vi "testing arm geometry.vi"(11 "arm angle (deg)":dbl(knob) min=-30.0 max=30.0 scale=30.0..-30.0) -> (1 "arm shuttle":cluster{"x":dbl, "y":dbl}={"x"=-9.11895003862225, "y"=13.0}, 3 "stroke max":dbl=17.75)   [LabVIEW 2020]
panel:
  out "angle (PI)":dbl=0.5 format="%.3g"
  out "In Range?":bool
  out "link to arm":cluster{"x":dbl, "y":dbl}={"x"=2.5000000000000004, "y"=16.0}
  out "hook ctr wrt CG":cluster{"x":dbl, "y":dbl}={"x"=4.000000000000003, "y"=46.25}
  in  "robot frame length (in)":dbl=30.0 format="%#_13g"
  in  "testing?":bool
  in  "hook outer diam (in)":dbl=4.0 format="%.3g"
  in  "coords to link (in)":cluster{"x":dbl, "y":dbl}[](array[cluster])=[{"x"=0.0, "y"=9.0}, {"x"=1.5, "y"=0.0}]
  in  "screw link (in)":dbl=12.0 format="%.3g"
  in  "stop":bool
  out "XY Graph":cluster{dbl[], dbl[]}[](graph)=[{[-31.0, -31.0, 31.0, 31.0], [0.0, 66.0, 66.0, 0.0]}, {[-29.0, -29.0, 29.0, 29.0], [0.0, 64.0, 64.0, 0.0]}, {[4.0, 4.000000000000003], [7.0, 46.25]}, {[2.5000000000000004, -9.11895003862225], [16.0, 13.0]}]
  in  "arm coords (in)":cluster{"x":dbl, "y":dbl}[](array[cluster])=[{"x"=0.0, "y"=32.5}, {"x"=0.0, "y"=3.0}, {"x"=0.0, "y"=3.75}]
  in  "screw pin AG (in)":dbl=13.0 format="%.3g"
  in  "shoulder pin back from CG (in)":dbl=4.0 format="%.3g"
  in  "shoulder pin AG (in)":dbl=7.0 format="%.3g"
  in  "Stroke (in)":dbl(slide) scale=0.0..23.0
  in  "height limit HANGAR (in)":dbl=66.0 format="%.3g"
  in  "frame reach limit (in)":dbl=16.0 format="%.3g"
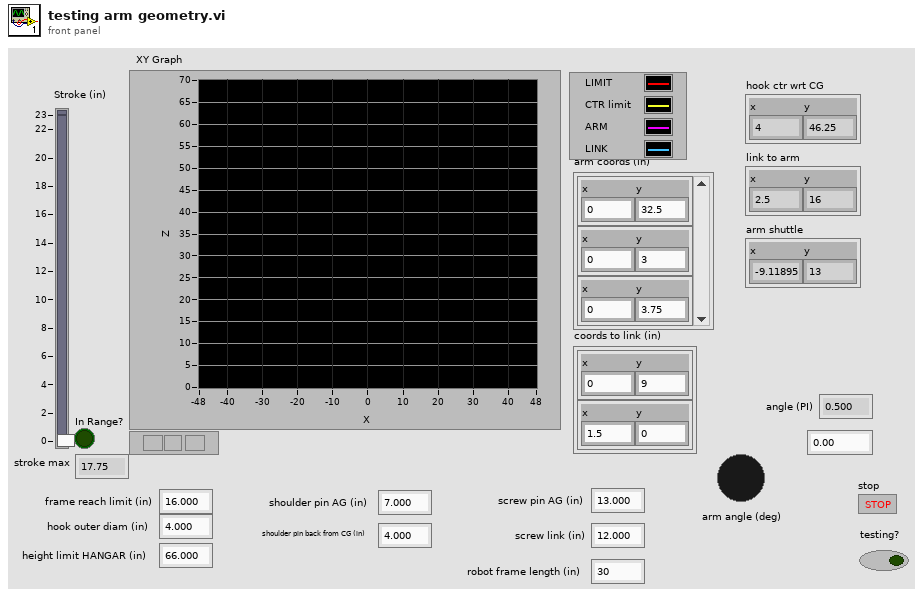
[diagram p1: front panel]
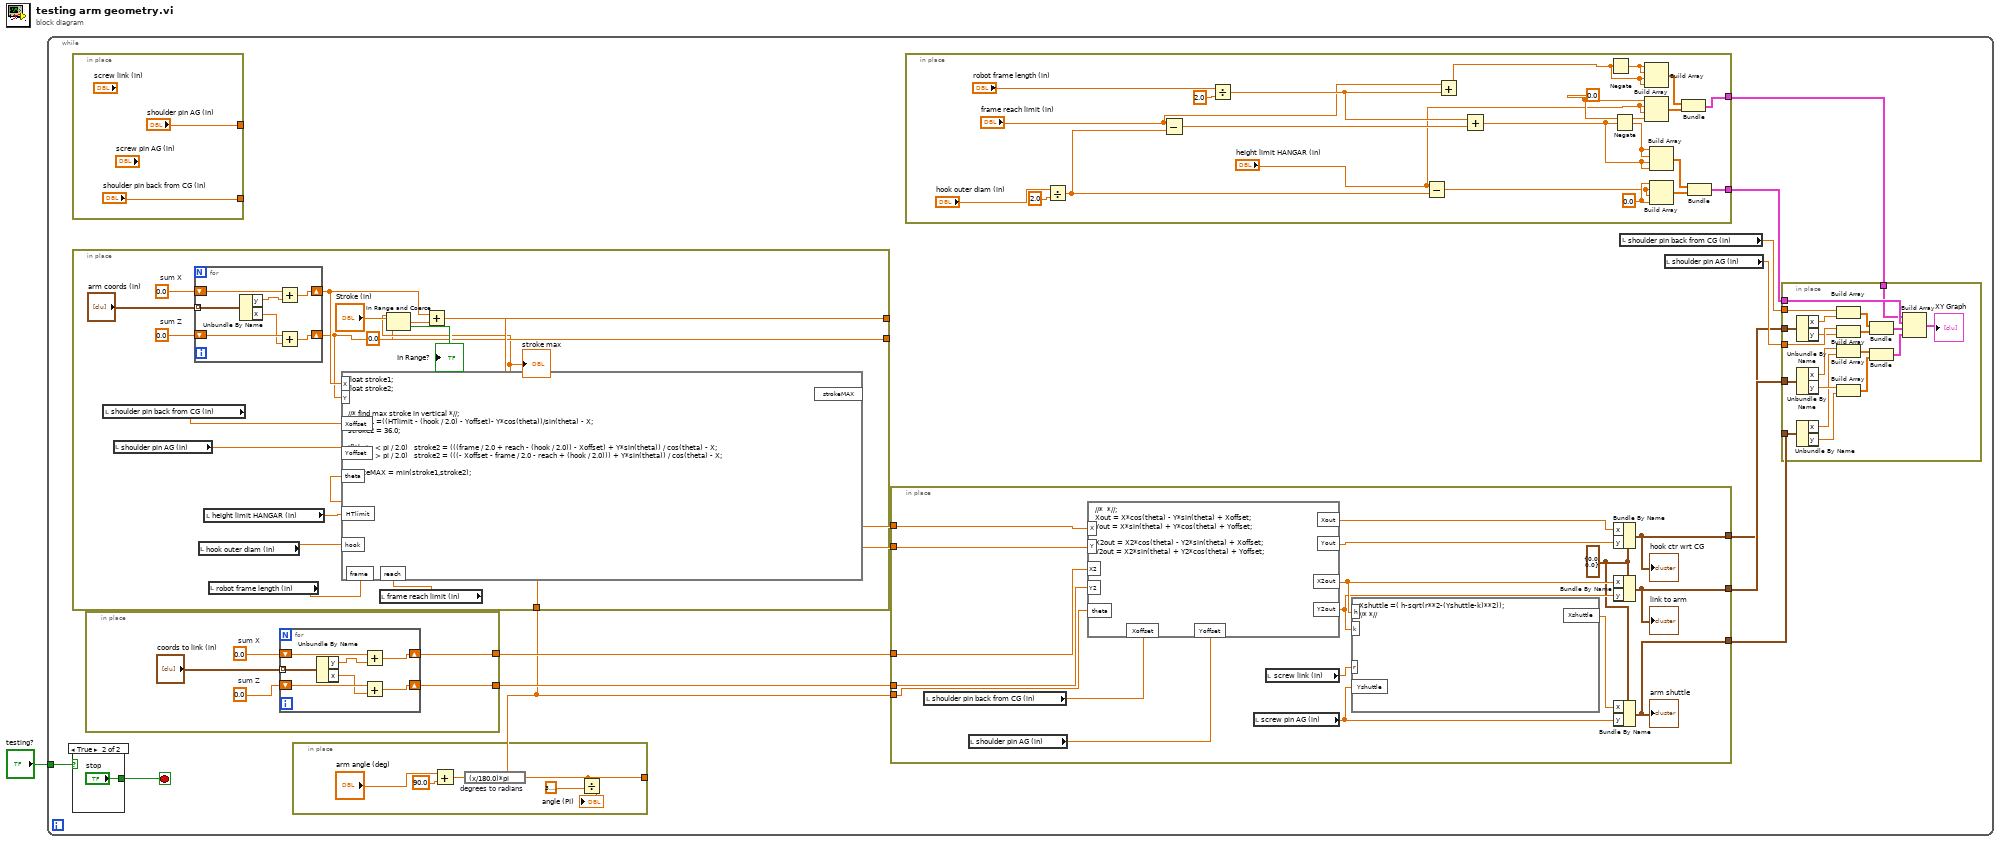
[diagram p0: block diagram]
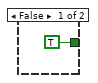
[diagram p2: hidden frame]
diagram:
  n1 = while {
    tunnel: "testing?" -> [w13]
    stop <- w15 stop-if-true
    n2 = in-place {
      in-place-border: ["shoulder pin back from CG (in)"] -> _
      in-place-border: ["shoulder pin AG (in)"] -> _
    }
    n3 = case shown="True" w13 {
      tunnel: [TRUE ("stop") "stop"] -> w15
      frame False {
      }
      frame True {
      }
    }
    n4 = in-place {
      in-place-border: [w64] -> w11
      in-place-border: [w62] -> w12
      w66 = 0.0  # sum X
      w65 = 0.0  # sum Z
      n5 = for {
        tunnel: "coords to link (in)" -> [w73] mode=indexing
        shift-right: [w71] -> w64
        shift-left: w65 -> [w72]
        shift-right: [w70] -> w62
        shift-left: w66 -> [w69]
        n6 = Unbundle By Name(w73) -> ("y"=w68:dbl, "x"=w67:dbl)
        n7 = Add(x=w69, y=w68) -> (x+y=w70:dbl)
        n8 = Add(x=w72, y=w67) -> (x+y=w71:dbl)
      }
    }
    n9 = in-place {
      in-place-border: [w41] -> w2
      n10 = Add(x="arm angle (deg)", y=90.0) -> (x+y=w38:dbl)
      n11 = expression code="(x/180.0)*pi" "degrees to radians"(w38) -> (w41:dbl)
      n12 = Divide(x=w41, y=3.141592653589793) -> (x/y=→"angle (PI)":dbl)
    }
    n13 = in-place {
      in-place-border: [w111] -> w10
      in-place-border: [w105] -> w9
      in-place-border: w2 -> [w103]
      w114 = 0.0  # sum X
      w113 = 0.0  # sum Z
      n14 = local read "shoulder pin back from CG (in)"() -> (w108:dbl)
      n15 = local read "shoulder pin AG (in)"() -> (w107:dbl)
      n16 = for {
        tunnel: "arm coords (in)" -> [w122] mode=indexing
        shift-right: [w120] -> w105
        shift-left: w113 -> [w121]
        shift-right: [w119] -> w106
        shift-left: w114 -> [w118]
        n17 = Unbundle By Name(w122) -> ("y"=w117:dbl, "x"=w116:dbl)
        n18 = Add(x=w118, y=w117) -> (x+y=w119:dbl)
        n19 = Add(x=w121, y=w116) -> (x+y=w120:dbl)
      }
      n20 = local read "hook outer diam (in)"() -> (w101:dbl)
      n21 = local read "height limit HANGAR (in)"() -> (w102:dbl)
      n22 = local read "robot frame length (in)"() -> (w98:dbl)
      n23 = local read "frame reach limit (in)"() -> (w99:dbl)
      n24 = formula code="float stroke1;\nfloat stroke2;\n\n\n//* find max stroke in vertical *//;\nstroke1 =((HTlimit - (hook / 2.0) - Yoffset)- Y*cos(theta))/sin(theta) - X;\nstroke2 = 36.0;\n\nif(theta < pi / 2.0)   stroke2 = (((frame / 2.0 + reach - (hook / 2.0)) - Xoffset) + Y*sin(theta)) / cos(theta) - X;\nif(theta > pi / 2.0)   stroke2 = (((- Xoffset - frame / 2.0 - reach + (hook / 2.0))) + Y*sin(theta)) / cos(theta) - X;\n\nstrokeMAX = min(stroke1,stroke2);"("Xoffset"=w108, "Yoffset"=w107, "theta"=w103, "X"=w106, "Y"=w105, "HTlimit"=w102, "hook"=w101, "frame"=w98, "reach"=w99) -> ("strokeMAX"=w104:dbl)
      "stroke max" <- w104
      n25 = In Range and Coerce(upper limit=w104, x="Stroke (in)", lower limit=0.0) -> (coerced(x)=w110:dbl, In Range?=→"In Range?":bool)
      n26 = Add(x=w106, y=w110) -> (x+y=w111:dbl)
    }
    n27 = in-place {
      in-place-border: w2 -> [w59]
      in-place-border: w12 -> [w56]
      in-place-border: w11 -> [w55]
      in-place-border: w10 -> [w54]
      in-place-border: w9 -> [w53]
      in-place-border: [w44] -> w6
      in-place-border: [w43] -> w5
      in-place-border: [w42] -> w4
      w45 = cluster{"x":dbl, "y":dbl} {"x"=0.0, "y"=0.0} ("Cluster")
      n28 = local read "shoulder pin back from CG (in)"() -> (w52:dbl)
      n29 = local read "shoulder pin AG (in)"() -> (w51:dbl)
      n30 = formula code="//*  *//;\nXout = X*cos(theta) - Y*sin(theta) + Xoffset;\nYout = X*sin(theta) + Y*cos(theta) + Yoffset;\n\nX2out = X2*cos(theta) - Y2*sin(theta) + Xoffset;\nY2out = X2*sin(theta) + Y2*cos(theta) + Yoffset;"("X"=w54, "Y"=w53, "theta"=w59, "X2"=w56, "Y2"=w55, "Xoffset"=w52, "Yoffset"=w51) -> ("Xout"=w58:dbl, "Yout"=w57:dbl, "X2out"=w50:dbl, "Y2out"=w49:dbl)
      n31 = local read "screw pin AG (in)"() -> (w46:dbl)
      n32 = local read "screw link (in)"() -> (w48:dbl)
      n33 = formula code="Xshuttle =( h-sqrt(r**2-(Yshuttle-k)**2));\n//* *//"("h"=w50, "k"=w49, "Yshuttle"=w46, "r"=w48) -> ("Xshuttle"=w47:dbl)
      n34 = Bundle By Name(cluster=w45, "x"=w58, "y"=w57) -> (w42:cluster{"x":dbl, "y":dbl})
      "hook ctr wrt CG" <- w42
      n35 = Bundle By Name(cluster=w45, "x"=w50, "y"=w49) -> (w43:cluster{"x":dbl, "y":dbl})
      "link to arm" <- w43
      n36 = Bundle By Name(cluster=w45, "x"=w47, "y"=w46) -> (w44:cluster{"x":dbl, "y":dbl})
      "arm shuttle" <- w44
    }
    n37 = in-place {
      in-place-border: [w88] -> w14
      in-place-border: [w74] -> w3
      w76 = 0.0 ("element")
      w89 = 0.0 ("element")
      n38 = Divide(x="hook outer diam (in)", y=2.0) -> (x/y=w83:dbl)
      n39 = Subtract(x="frame reach limit (in)", y=w83) -> (x-y=w87:dbl)
      n40 = Divide(x="robot frame length (in)", y=2.0) -> (x/y=w80:dbl)
      n41 = Subtract(x="height limit HANGAR (in)", y=w83) -> (x-y=w84:dbl)
      n42 = Add(x="frame reach limit (in)", y=w80) -> (x+y=w78:dbl)
      n43 = Add(x=w80, y=w87) -> (x+y=w90:dbl)
      n44 = Negate(x=w78) -> (-x=w77:dbl)
      n45 = Negate(x=w90) -> (-x=w91:dbl)
      n46 = Build Array(w77, w77, w78, w78) -> (w81:dbl[])
      n47 = Build Array(w76, "height limit HANGAR (in)", "height limit HANGAR (in)", w76) -> (w82:dbl[])
      n48 = Build Array(w91, w91, w90, w90) -> (w94:dbl[])
      n49 = Build Array(w89, w84, w84, w89) -> (w95:dbl[])
      n50 = Bundle(w81, w82) -> (w74:cluster{dbl[], dbl[]})  [unwired: 1 in]
      n51 = Bundle(w94, w95) -> (w88:cluster{dbl[], dbl[]})  [unwired: 1 in]
    }
    n52 = local read "shoulder pin back from CG (in)"() -> (w7:dbl)
    n53 = local read "shoulder pin AG (in)"() -> (w8:dbl)
    n54 = in-place {
      in-place-border: w14 -> [w31]
      in-place-border: w7 -> [w27]
      in-place-border: w8 -> [w26]
      in-place-border: w6 -> [w22]
      in-place-border: w5 -> [w25]
      in-place-border: w4 -> [w19]
      in-place-border: w3 -> [w16]
      n55 = Unbundle By Name(w19) -> ("x"=w18:dbl, "y"=w17:dbl)
      n56 = Unbundle By Name(w25) -> ("x"=w24:dbl, "y"=w23:dbl)
      n57 = Unbundle By Name(w22) -> ("x"=w20:dbl, "y"=w21:dbl)
      n58 = Build Array(w27, w18) -> (w34:dbl[])
      n59 = Build Array(w26, w17) -> (w35:dbl[])
      n60 = Build Array(w24, w20) -> (w29:dbl[])
      n61 = Build Array(w23, w21) -> (w30:dbl[])
      n62 = Bundle(w34, w35) -> (w32:cluster{dbl[], dbl[]})  [unwired: 1 in]
      n63 = Bundle(w29, w30) -> (w28:cluster{dbl[], dbl[]})  [unwired: 1 in]
      n64 = Build Array(w16, w31, w32, w28) -> (→"XY Graph":cluster{dbl[], dbl[]}[])
    }
  }
